vi "SetAzCamToolParameter.vi"(1 "Value":string, 2 "Parameter":string) -> (0 "Error":bool)   [LabVIEW 2014]
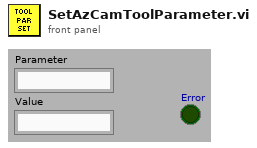
[diagram p1: front panel]
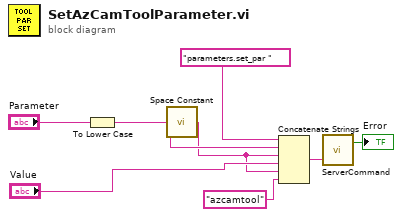
[diagram p0: block diagram]
diagram:
  n1 = To Lower Case(string="Parameter") -> (all lower case string=w4:string)
  n2 = call <vilib>:"Space Constant.vi"() -> ("String"=w1:string)
  n3 = Concatenate Strings("parameters.set_par " ("Attribute"), w4, w1, "Value", w1, "azcamtool" ("Attribute")) -> (w8:string)
  n4 = call "ServerCommand.vi"("Command"=w8) -> ("Error"=→"Error":bool)  [unwired: 1 out]
